vi "Detailed Data.vi"(11 "Data":T1) -> ()   [LabVIEW 2025, in "Full User Interface.lvlib"]
uses:
  Full User Interface.lvlib
panel:
  in  "Multicolumn Listbox":i32(listbox)
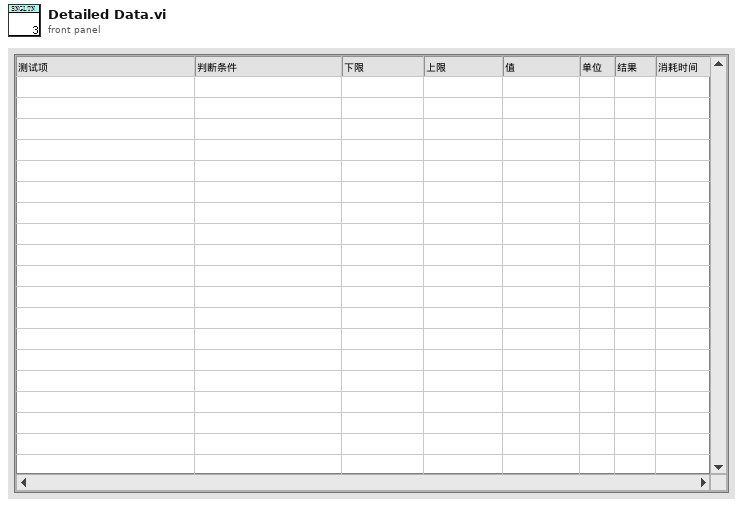
[diagram p1: front panel]
types:
  T1 = cluster{"Cluster":cluster{"General":cluster{"Sequence Name":string, "Serial Number":string, "Test Date Time":string, "UUT Status":string, "Faulty Item":string, "Seconds Executing":string}, "Tree Control Items":cluster{"Left Cell String":string, "Child Text":string[], "Child Tag":string, "Item Indent":i32, "Child Only?":bool, "Glyph Index":i32}[]}, "Station":string, "Socket":i32}
  T2 = cluster{"Left Cell String":string, "Child Text":string[], "Child Tag":string, "Item Indent":i32, "Child Only?":bool, "Glyph Index":i32}[]
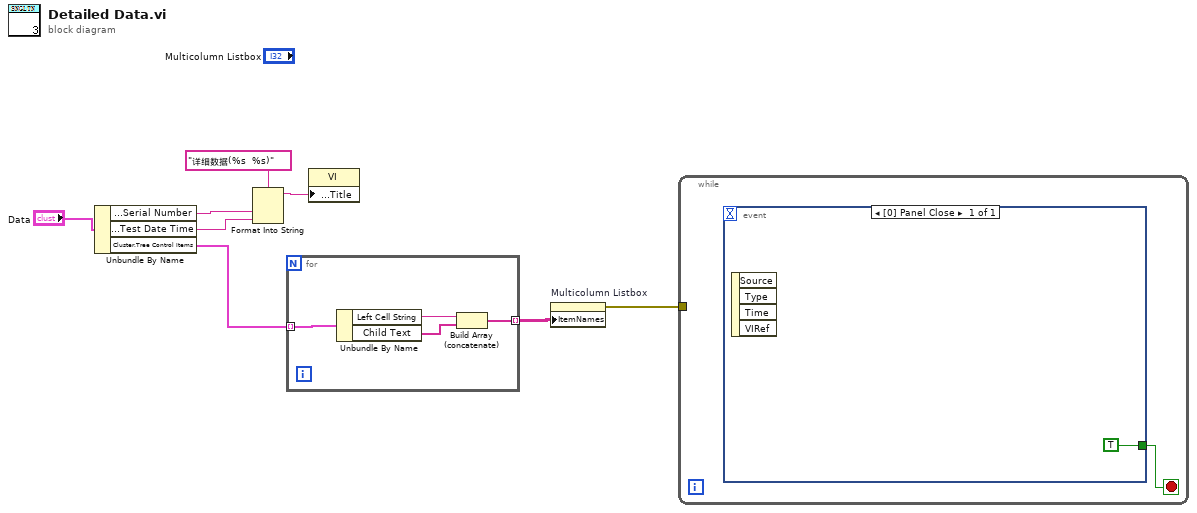
[diagram p0: block diagram]
diagram:
  n1 = Unbundle By Name("Data") -> ("Cluster.General.Serial Number"=w6:string, "Cluster.General.Test Date Time"=w5:string, "Cluster.Tree Control Items"=w3:T2)
  n2 = Format Into String(format string="详细数据(%s  %s)", w6, w5) -> (resulting string=w4:string)  [unwired: 2 in, 1 out]
  n3 = for {
    tunnel: w3 -> [w12] mode=indexing
    tunnel: [w9] -> w2 mode=indexing
    n4 = Unbundle By Name(w12) -> ("Left Cell String"=w11:string, "Child Text"=w10:string[])
    n5 = Build Array (concatenate)(w11, w10) -> (w9:string[])
  }
  n6 = property class="VI"("Front Panel.Title"=w4) -> ()  [unwired: 2 in, 2 out]
  n7 = property on="Multicolumn Listbox" class="MCListbox (strict)"("ItemNames"=w2) -> (error out=w1:errorcluster)  [unwired: 2 in, 1 out]
  n8 = while {
    tunnel: w1 -> [_]
    stop <- w13 stop-if-true
    n9 = event shown="[0] Panel Close" {
      selector: _ -> [_]
      dyn-events: _ -> [_]
      timeout: _ -> [_]
      tunnel: [TRUE] -> w13
      event Panel Close {
        n10 = event-data() -> ()  [unwired: 1 in, 4 out]
      }
    }
  }
